vi "all_tests.vi"() -> ()   [LabVIEW 2020]
panel:
  in  "error in":errorcluster
  out "error out":errorcluster
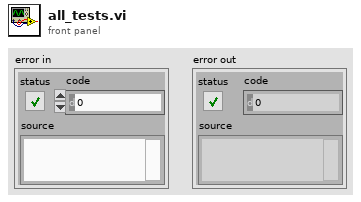
[diagram p1: front panel]
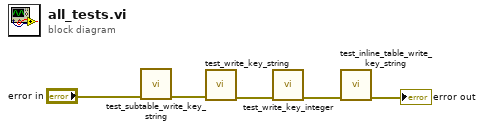
[diagram p0: block diagram]
diagram:
  n1 = call "test_subtable_write_key_string.vi"("error in (no error)"="error in") -> ("error out"=w4:errorcluster)  [unwired: 10 in]
  n2 = call "test_write_key_string.vi"("error in (no error)"=w4) -> ("error out"=w5:errorcluster)  [unwired: 10 in]
  n3 = call "test_write_key_integer.vi"("error in (no error)"=w5) -> ("error out"=w2:errorcluster)  [unwired: 10 in]
  n4 = call "test_inline_table_write_key_string.vi"("error in (no error)"=w2) -> ("error out"=→"error out":errorcluster)  [unwired: 10 in]
